vi "Klinger AxisParams.vi"(0 "Axe":u8(ring) items=["W", "X", "Y", "Z"], 1 "TypeMouv":i32(ring) caption="Type de mouvement" items=["Linéaire", "Rotation"], 2 "Nom de l'axe":string, 5 "Type":i32(ring) caption="Type de moteur" items=["UE30", "UE72"], 7 "FactConv":dbl=0.01 caption="Facteur de\nConversion\n(m/pas ou °/pas)", 9 "CorrParams":T1={"CorrActive"=FALSE, "ErreurLim"=0.1, "NbrEssais"=3} caption="Paramètres de correction de position" {"NbrEssais" min=1 max=5 step=1; "ErreurLim" min=0.0 max=10.0 step=0.1 format="%#.1f"}, 11 "error in":errorcluster, 12 "Encodeur":bool caption="Possède un\nEncodeur", 13 "MiseàZéro":bool caption="Possède un\nInterrupteur d'origine") -> (15 "error out":errorcluster)   [LabVIEW 2010]
doc: "Ce Vi de lire et d'écrire les paramètres des différents axes du fichier .ini"
panel:
  in  "Quitter":bool
  in  "Save":bool
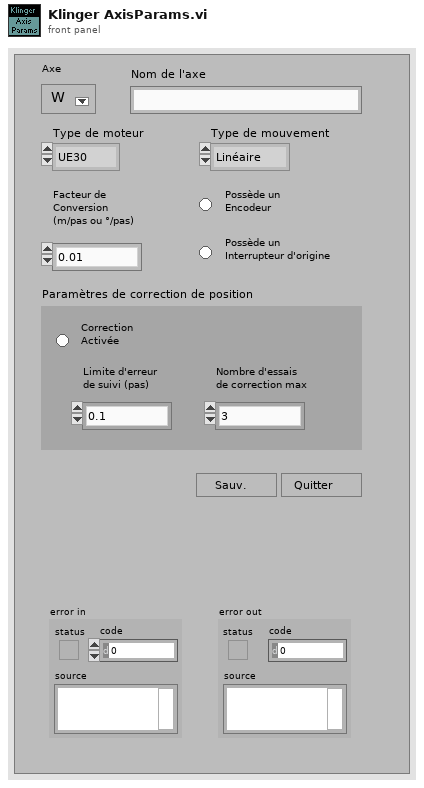
[diagram p1: front panel]
types:
  T1 = cluster{"CorrActive":bool, "ErreurLim":dbl, "NbrEssais":i32}
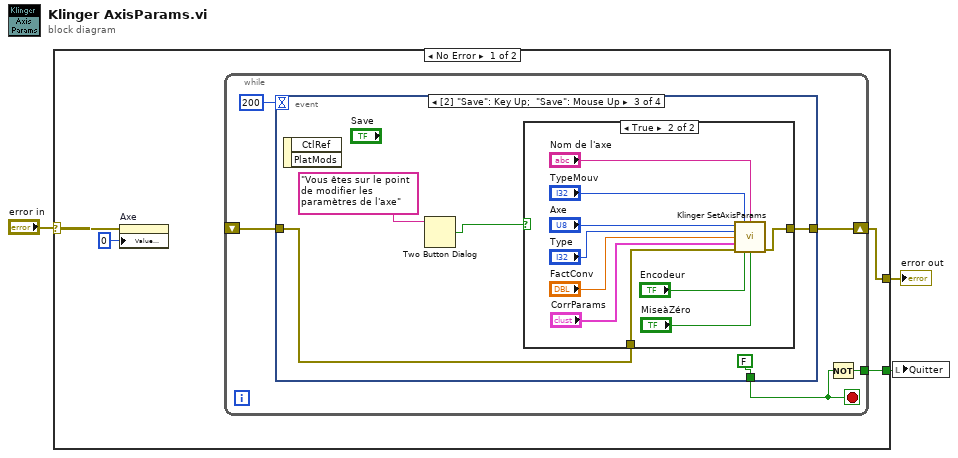
[diagram p0: block diagram]
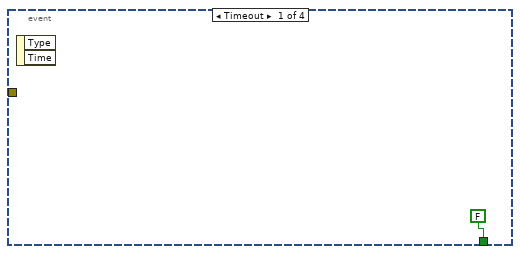
[diagram p2: hidden frame]
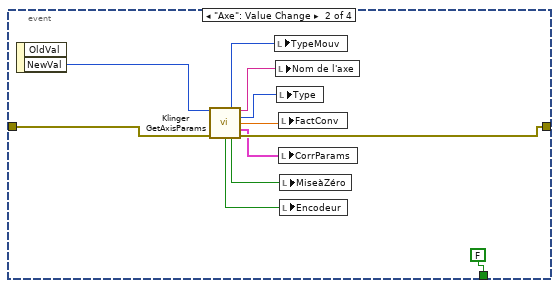
[diagram p3: hidden frame]
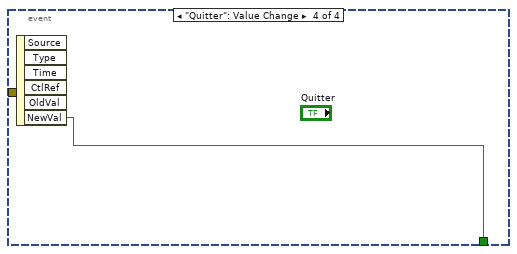
[diagram p5: hidden frame]
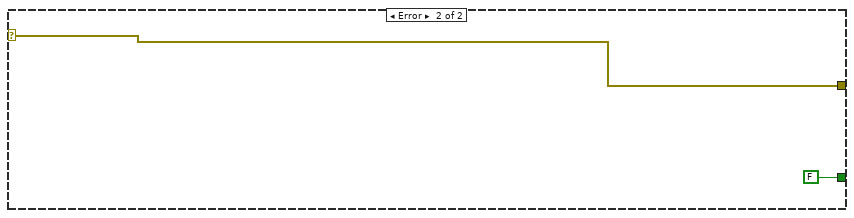
[diagram p6: hidden frame]
diagram:
  n1 = case shown="No Error" "error in" {
    selector: "error in" -> [w5 w43]
    tunnel: [w7 w43] -> w3
    tunnel: [w4 FALSE] -> w1
    frame No Error {
      n2 = property on="Axe" class="Ring (strict)"(error in=w5, "Value (Signaling)"=u8 0) -> ()  [unwired: 1 in, 2 out]
      n3 = while {
        shift-right: [w10] -> w7
        shift-left: _ -> [w11]
        tunnel: [w8] -> w4
        stop <- w9 stop-if-true
        n4 = event shown="[2] \"Save\": Key Up;  \"Save\": Mouse Up" {
          selector: _ -> [_ _ _ _]
          dyn-events: _ -> [_ _ _ _]
          timeout: 200 -> [_ _ _ _]
          tunnel: [FALSE FALSE FALSE w41] -> w9
          tunnel: w11 -> [_ w22 w28 _]
          tunnel: [_ w21 w27 _] -> w10
          event Timeout {
            n5 = event-data() -> ()  [unwired: 1 in, 2 out]
          }
          event "Axe": Value Change {
            n6 = event-data() -> ("NewVal"=w23:u8)  [unwired: 1 in, 1 out]
            n7 = call <userlib>:"Klinger GetAxisParams.vi"("Axe"=w23, "error in"=w22) -> ("TypeMouv"=w20:i32, "Nom de l'axe"=w19:string, "Type"=w18:i32, "FactConv"=w17:dbl, "CorrParams"=w16:T1, "Encodeur"=w14:bool, "MiseàZéro"=w15:bool, "error out"=w21:errorcluster)  [unwired: 6 in]
            n8 = local write "TypeMouv"(w20) -> ()
            n9 = local write "Nom de l'axe"(w19) -> ()
            n10 = local write "Type"(w18) -> ()
            n11 = local write "FactConv"(w17) -> ()
            n12 = local write "CorrParams"(w16) -> ()
            n13 = local write "MiseàZéro"(w15) -> ()
            n14 = local write "Encodeur"(w14) -> ()
          }
          event "Save": Key Up; "Save": Mouse Up {
            n15 = event-data() -> ()  [unwired: 1 in, 2 out]
            n16 = Two Button Dialog(message="Vous êtes sur le point de modifier les paramètres de l'axe") -> (T button?=w25:bool)  [unwired: 2 in]
            n17 = case shown="True" w25 {
              tunnel: w28 -> [w30 w35]
              tunnel: [w30 w33] -> w27
              frame False {
              }
              frame True {
                n18 = call <userlib>:"Klinger SetAxisParams.vi"("Axe"="Axe", "TypeMouv"="TypeMouv", "Nom de l'axe"="Nom de l'axe", "Type"="Type", "FactConv"="FactConv", "CorrParams"="CorrParams", "error in"=w35, "Encodeur"="Encodeur", "MiseàZéro"="MiseàZéro") -> ("error out"=w33:errorcluster)  [unwired: 6 in]
              }
            }
          }
          event "Quitter": Value Change {
            n19 = event-data() -> ("NewVal"=w41:bool)  [unwired: 1 in, 5 out]
          }
        }
        n20 = Not(x=w9) -> (.not. x?=w8:bool)
      }
    }
    frame Error {
    }
  }
  "error out" <- w3
  n21 = local write "Quitter"(w1) -> ()
